vi "InitSubRTM.vi"(8 "error in (no error)":errorcluster, 9 "RTM Path":path, 10 "CtrlRef":refnum<vi>, 11 "Menu in":refnum<class "Menu.lvclass">) -> (0 "error out":errorcluster, 2 "MenuSelectionEvent":refnum<user-event>, 3 "Menu out":refnum<class "Menu.lvclass">)   [LabVIEW 2021, in "Menu.lvlib" / "Menu.lvclass"]
uses:
  Menu.lvclass
  MenuSelection.ctl
  Data.ctl
  MenuItems.ctl
  <vilib>/Utility/miscctls.llb/LVMenuShortCut.ctl
  Picture2D/src/Picture/Image.lvclass
  TD_CloseEvent.ctl
  MenuColors.ctl
  Picture2D/src/Color/Color.lvclass
  Picture2D/src/Font/Font.lvclass
  SubMenuIcon.ctl
  Picture2D/src/Picture2D/Picture2D.lvclass
  Menu.lvclass/Menu.ctl
  TR_ManageContextMenu.vi
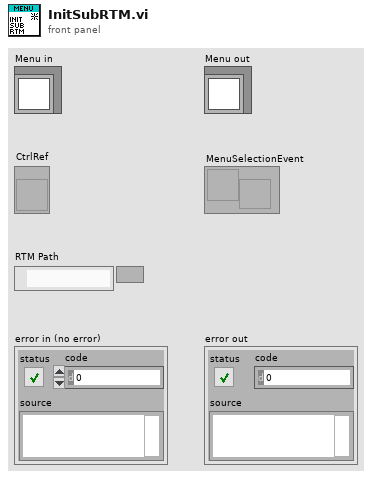
[diagram p1: front panel]
types:
  T1 = typedef "Menu.lvlib/Menu.lvclass/MenuSelection.ctl" = cluster{"ItemTag":string, "ItemPath":string}
  T2 = typedef "Menu.lvlib/Menu.lvclass/TD_CloseEvent.ctl" = cluster{"Close":bool}
  T3 = typedef "Menu.lvlib/Menu.lvclass/Data.ctl" = cluster{"MenuMap":map{string, T4}, "PictRef":refnum<vi>, "MenuSelectionEvent":refnum<user-event>, "TopMenuSpacing":i32, "MenuSpacing":i32, "CloseEvent":refnum<user-event>, "TR_ManageMenuRef":refnum<vi>, "MenuColors":T6, "RTMPath":path, "RTMVIReference":refnum<vi>, "RTMMenuReference":refnum<k9>, "CtlRef":refnum<vi>, "User-Specified Font":refnum<class "Font.lvclass">, "Desired Font":enum16{"User-specified Font", "Application Font", "System Font", "Dialog Font"}, "SubMenuIcon":T7, "SubMenuIconClosed":refnum<class "Picture2D.lvclass">, "SubMenuIconOpened":refnum<class "Picture2D.lvclass">}
  T4 = typedef "Menu.lvlib/Menu.lvclass/MenuItems.ctl" = cluster{"Item Name":string, "Short Cut":T5, "Checked":bool, "Enable":bool, "After item":string, "Item Tags":string[], "Item Names":string[], "Picture":refnum<class "Image.lvclass">, "Hilite Picture":refnum<class "Image.lvclass">, "Displayed":bool}
  T5 = typedef "LVMenuShortCut.ctl" = cluster{"Include Shift Key?":bool, "Include Ctrl Key?":bool, "Shortcut Key":string}
  T6 = typedef "Menu.lvlib/Menu.lvclass/MenuColors.ctl" = cluster{"Text":refnum<class "Color.lvclass">, "HiliteText":refnum<class "Color.lvclass">, "Background":refnum<class "Color.lvclass">, "BorderColor":refnum<class "Color.lvclass">, "Hilite":refnum<class "Color.lvclass">}
  T7 = typedef "Menu.lvlib/Menu.lvclass/SubMenuIcon.ctl" = enum16{"LabVIEW", "Windows", "Custom"}
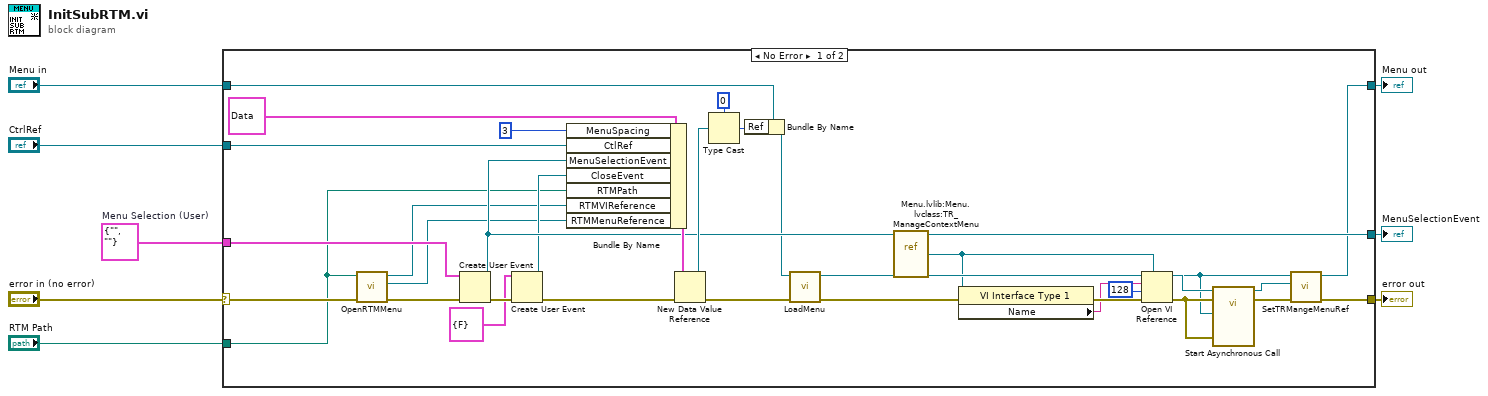
[diagram p0: block diagram]
diagram:
  w6 = T1 {"ItemTag"="", "ItemPath"=""}  # Menu Selection (User)
  n1 = case shown="No Error" "error in (no error)" {
    selector: "error in (no error)" -> [w17 w42]
    tunnel: "CtrlRef" -> [w36 _]
    tunnel: w6 -> [w35 _]
    tunnel: [w34 _] -> w5
    tunnel: "Menu in" -> [w24 w43]
    tunnel: [w22 w42] -> w3
    tunnel: [w20 w43] -> w2
    tunnel: "RTM Path" -> [w15 _]
    frame No Error {
      n2 = call "OpenRTMMenu.vi"("error in"=w17, "RTMFilePath"=w15) -> ("error out"=w16:errorcluster, "RTMMenuReference"=w13:refnum<k9>, "RTMVIReference"=w14:refnum<vi>)  [unwired: 7 in]
      n3 = Create User Event(user event datatype=w35, error in=w16) -> (user event=w34:refnum<user-event>, error out=w27:errorcluster)
      n4 = Create User Event(user event datatype=T2 {"Close"=FALSE} ("CloseEvent"), error in=w27) -> (user event=w25:refnum<user-event>, error out=w26:errorcluster)
      n5 = Bundle By Name(cluster=T3 {"MenuMap"={}, "PictRef"=refnum, "MenuSelectionEvent"=refnum, "TopMenuSpacing"=0, "MenuSpacing"=0, "CloseEvent"=refnum, "TR_ManageMenuRef"=refnum, "MenuColors"={"Text"=refnum, "HiliteText"=refnum, "Background"=refnum, "BorderColor"=refnum, "Hilite"=refnum}, "RTMPath"=path "", "RTMVIReference"=refnum, "RTMMenuReference"=refnum, "CtlRef"=refnum, "User-Specified Font"=refnum, "Desired Font"=enum."User-specified Font", "SubMenuIcon"=enum."LabVIEW", "SubMenuIconClosed"=refnum, "SubMenuIconOpened"=refnum} ("Data"), "MenuSpacing"=3, "CtlRef"=w36, "MenuSelectionEvent"=w34, "CloseEvent"=w25, "RTMPath"=w15, "RTMVIReference"=w14, "RTMMenuReference"=w13) -> (w37:T3)
      n6 = New Data Value Reference(data value=w37, error in=w26) -> (data value reference=w39:refnum<data-value>, error out=w30:errorcluster)
      n7 = Type Cast(type=u64 0 ("Ref"), x=w39) -> (*(type *) &x=w41:u64)
      n8 = Bundle By Name(cluster=w24, "Ref"=w41) -> (w21:refnum<class "Menu.lvclass">)
      n9 = call "LoadMenu.vi"("error in (no error)"=w30, "Menu in"=w21) -> ("error out"=w11:errorcluster, "Menu out"=w10:refnum<class "Menu.lvclass">)  [unwired: 8 in]
      n10 = vi-ref "Menu.lvlib:Menu.lvclass:TR_ManageContextMenu.vi"() -> (w9:refnum<vi>)
      n11 = property class="VI Interface Type 1"(reference=w9, error in=w11) -> (error out=w32:errorcluster, "Name"=w29:string)  [unwired: 1 out]
      n12 = Open VI Reference(type specifier VI Refnum (for type only)=w9, vi path=w29, options=128, error in (no error)=w32) -> (vi reference=w33:refnum<vi>, error out=w28:errorcluster)  [unwired: 2 in]
      n13 = call-by-ref "Start Asynchronous Call"(reference=w33, error in=w28, 8:"error in (no error)"=w28, "Menu in"=w10) -> (reference out=w19:refnum<vi>, error out=w23:errorcluster)  [unwired: 9 in, 1 out]
      n14 = call "SetTRMangeMenuRef.vi"("error in (no error)"=w23, "TR_ManageMenuRef"=w19, "Menu in"=w10) -> ("error out"=w22:errorcluster, "Menu out"=w20:refnum<class "Menu.lvclass">)  [unwired: 7 in]
    }
    frame Error {
    }
  }
  "error out" <- w3
  "Menu out" <- w2
  "MenuSelectionEvent" <- w5
